vi "calculate drive to peg.vi"(0 "status":dbl, 1 "center x (0-319)":dbl, 2 "size x (1-320)":dbl) -> (7 "x":dbl, 9 "y":dbl)   [LabVIEW 2016]
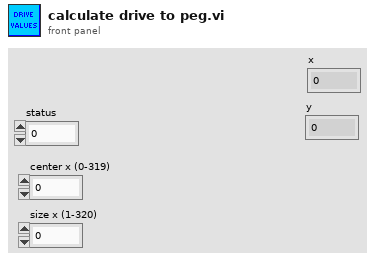
[diagram p1: front panel]
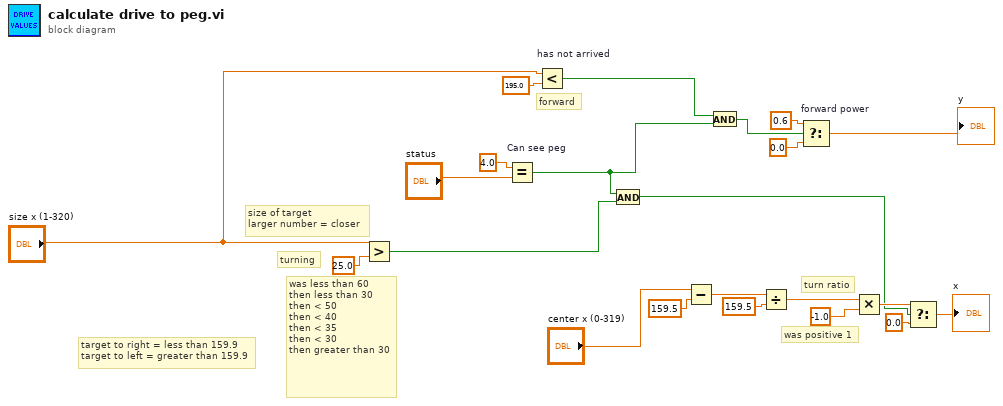
[diagram p0: block diagram]
diagram:
  # "forward"
  # "was positive 1"
  # "turning"
  # "size of target\nlarger number = closer"
  # "turn ratio"
  # "was less than 60\nthen less than 30\nthen < 50\nthen < 40\nthen < 35\nthen < 30\nthen greater than 30"
  # "target to right = less than 159.9\ntarget to left = greater than 159.9"
  n1 = Greater?(x="size x (1-320)", y=25.0) -> (0:w9:bool)
  n2 = Equal? "Can see peg"(x=4.0 ("y"), y="status") -> (x = y?=w7:bool)
  n3 = Less? "has not arrived"(x="size x (1-320)", y=195.0) -> (x < y?=w8:bool)
  n4 = And(x=w7, y=w9) -> (x .and. y?=w12:bool)
  n5 = Subtract(x="center x (0-319)", y=159.5) -> (x-y=w18:dbl)
  n6 = And(x=w8, y=w7) -> (x .and. y?=w11:bool)
  n7 = Divide(x=w18, y=159.5) -> (x/y=w14:dbl)
  n8 = Select "forward power"(t=0.6, s=w11, f=0.0) -> (s? t:f=→"y":dbl)
  n9 = Multiply(x=w14, y=-1.0) -> (x*y=w15:dbl)
  n10 = Select(t=w15, s=w12, f=0.0) -> (s? t:f=→"x":dbl)
